vi "TesterCode.vi"() -> ()   [LabVIEW 2019]
uses:
  <vilib>/picture/picture.llb/imagedata.ctl
  Histograph.ctl
panel:
  out "Histogram Graph":T1
  out "Most likely":cluster{"score":dbl, "class":string}[](array[cluster])
  out "Intensity Graph":u8[][](graph)
  out "Grey":T2
  out "Blue":T2
  out "Green":T2
  out "Red":T2
  out "new picture":picture
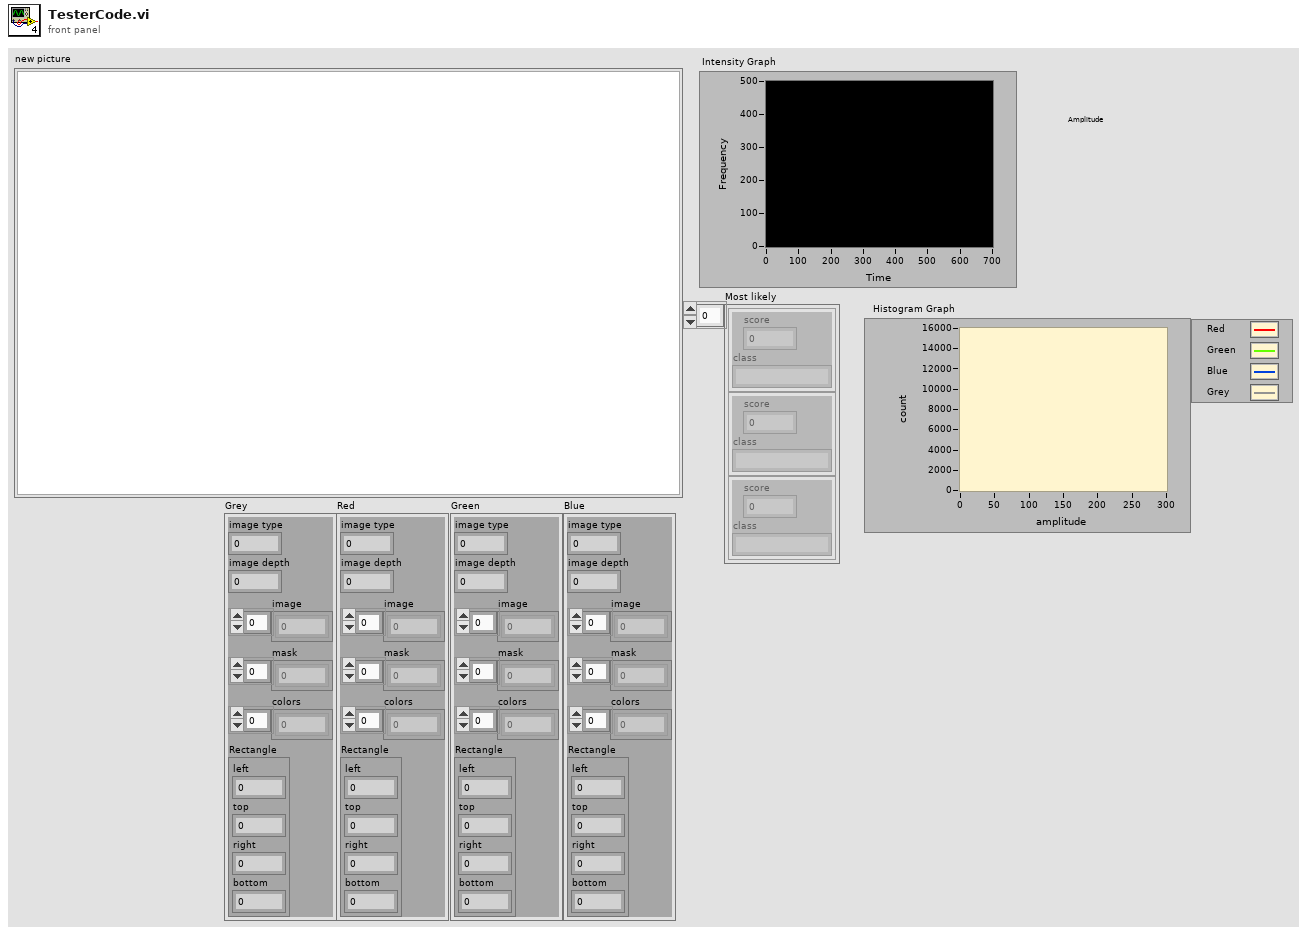
[diagram p1: front panel]
types:
  T1 = typedef "Histograph.ctl" = cluster{"X Values":dbl[], "Histogram: h(x)":i32[]}[]
  T2 = typedef "imagedata.ctl" = cluster{"image type":i32, "image depth":i32, "image":u8[], "mask":u8[], "colors":u32[], "Rectangle":cluster{"left":i16, "top":i16, "right":i16, "bottom":i16}}
  T3 = enum16{"No Change", "Apricot", "Carnation", "Ether", "Greyscale", "Greyscale-banded", "Hot Metal", "Lava Waves", "Mac", "Morning Glory", "Rainbow", "Rainbow-banded", "Rainbow-inverted", "Rainbow-striped", "Saturn", "Seismic", "Space"}
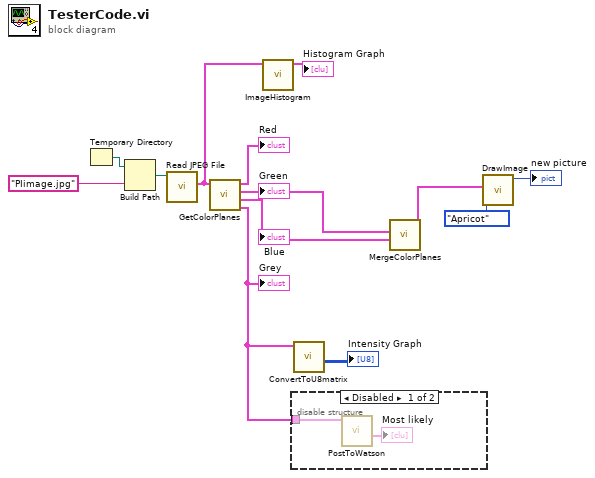
[diagram p0: block diagram]
diagram:
  n1 = Temporary Directory() -> (w13:path)
  n2 = Build Path(base path=w13, name or relative path="PIimage.jpg") -> (appended path=w11:path)
  n3 = call <vilib>:"Read JPEG File.vi"("path to JPEG file"=w11) -> ("image data"=w5:T2)  [unwired: 8 in, 2 out]
  n4 = call "GetColorPlanes.vi"("image data"=w5) -> ("Grey"=w8:T2, "Blue"=w3:T2, "Green"=w4:T2, "Red"=→"Red":T2)  [unwired: 7 in]
  "Green" <- w4
  "Blue" <- w3
  "Grey" <- w8
  n5 = call "ImageHistogram.vi"("image data"=w5) -> ("Histogram Graph"=→"Histogram Graph":T1)  [unwired: 10 in]
  n6 = disable-structure shown="Disabled" {
    disable-tunnel: w8 -> [w15 _]
    frame Disabled {
      n7 = call "PostToWatson.vi"("image in"=w15) -> ("Most likely"=→"Most likely":cluster{"score":dbl, "class":string}[])  [unwired: 6 in, 4 out]
    }
    frame Enabled {
    }
  }
  n8 = call "ConvertToU8matrix.vi"("Image In"=w8) -> ("Intensity Graph"=→"Intensity Graph":u8[][])  [unwired: 9 in, 1 out]
  n9 = call "MergeColorPlanes.vi"("Blue"=w3, "Green"=w4) -> ("image data"=w2:T2)  [unwired: 9 in]
  n10 = call "DrawImage.vi"("Color Table"=T3."Apricot", "Image In"=w2) -> ("new picture"=→"new picture":picture)  [unwired: 9 in]
